vi "Remove.vi"(8 "error in (no error)":errorcluster, 11 "input in":refnum<class "Input.lvclass">) -> (0 "error out":errorcluster, 3 "input out":refnum<class "Input.lvclass">)   [LabVIEW 2015, in "Input.lvclass"]
uses:
  Input.lvclass
  Input.lvclass/Input.ctl
  <vilib>/ActorFramework/Message Enqueuer/Message Enqueuer.lvclass/Message Enqueuer.ctl
  <vilib>/ActorFramework/Message Enqueuer/Enqueue.vi
  <vilib>/ActorFramework/Message Priority Queue/Priority Enqueue.vi
  <vilib>/ActorFramework/Stop Msg/Stop Msg.lvclass
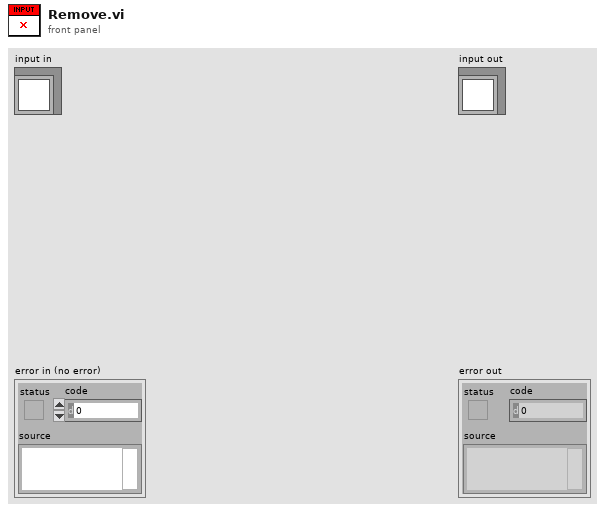
[diagram p1: front panel]
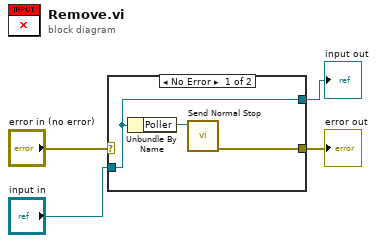
[diagram p0: block diagram]
diagram:
  n1 = case shown="No Error" "error in (no error)" {
    selector: "error in (no error)" -> [_ w9]
    tunnel: [w5 w9] -> w3
    tunnel: [w7 w8] -> w1
    tunnel: "input in" -> [w7 w8]
    frame No Error {
      n2 = Unbundle By Name(w7) -> ("Poller"=w6:refnum<class "Message Enqueuer.lvclass">)
      n3 = call <vilib>:"Send Normal Stop.vi"("Message Enqueuer"=w6) -> ("error out"=w5:errorcluster)  [unwired: 10 in]
    }
    frame Error {
    }
  }
  "error out" <- w3
  "input out" <- w1
